vi "Read myBool.vi"(8 "error in (no error)":errorcluster, 11 "Class2 in":refnum<class "Class2.lvclass">) -> (0 "error out":errorcluster, 2 "myBool":bool, 3 "Class2 out":refnum<class "Class2.lvclass">)   [LabVIEW 2020, in "Class2.lvclass"]
doc: "GCraftsman JSON Object Serialization Toolkit\nwww.GCraftsman.com\nCopyright (c) 2017, GCraftsman"
uses:
  Class2.lvclass
  Class2.lvclass/Class2.ctl
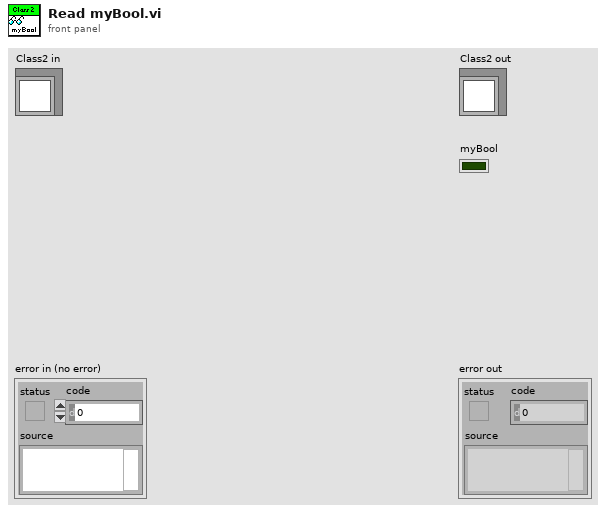
[diagram p1: front panel]
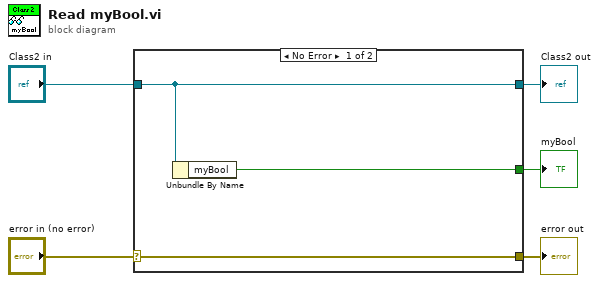
[diagram p0: block diagram]
diagram:
  n1 = case shown="No Error" "error in (no error)" {
    selector: "error in (no error)" -> [w8 w9]
    tunnel: [w8 w9] -> w4
    tunnel: [w7 w10] -> w2
    tunnel: "Class2 in" -> [w7 w10]
    tunnel: [w6 _] -> w1
    frame No Error {
      n2 = Unbundle By Name(w7) -> ("myBool"=w6:bool)
    }
    frame Error {
    }
  }
  "error out" <- w4
  "Class2 out" <- w2
  "myBool" <- w1
